vi "MAIN_red.vi"() -> ()   [LabVIEW 2011]
uses:
  <vilib>/event_ctls.llb/eventsource.ctl
  <vilib>/userDefined/High Color/IMAQdx.ctl
  <vilib>/vision/driver/NI_Vision_Acquisition_Software.lvlib
  <vilib>/vision/NI_Vision_Development_Module.lvlib
panel:
  in  "Session In":T1="BW14bits Focused"
  out "X position":dbl
  out "Y position 1":dbl
  out "Y position 2":dbl
  out "X 2":dbl
  out "Source":T2 items=["LabVIEW UI"=0, "ActiveX"=1, "User Event"=25]
  in  "Save":bool
  in  "Color":bool
  out "Image":T3(plugin-control)
  out "Histograph":T4(graph)={"Starting Value"=-32768.0, "Incremental Value"=1.0, "Histogram"=array[65536 elements]}
  out "# Sat. Pixels":sgl(slide) scale=0.0..5000.0
  out "error out 4":errorcluster
  in  "SLM 2":enum32{"Viewer & Positioner", "Hologram Loader"}(tab)
  out "<< CGH_y\n      SLM 2":T3(plugin-control)
  in  "X position 2":dbl(slide)=5.082508250825082 scale=0.0..10.0
  in  "Fine:":dbl(slide)=4.934210526315789 scale=0.0..10.0
  in  "Fine:":dbl(slide)=4.883720930232558 scale=0.0..10.0
  in  "Y position 3":dbl(slide)=4.883720930232558 scale=0.0..10.0
  out "String 2":string
  in  "Xoffset2":dbl=-1325.0
  in  "Yoffset2":dbl=-225.0
  out "String 3":string
  out "SLM 3":T3(plugin-control)
  in  "Radio Buttons":T5(radio)=enum."Radio Selection 2"
  in  "Semi2":bool caption="Boolean"
  in  "Phase correction 2":bool
  in  "M4":bool
  in  "Holo:":dbl=1.0
  out "Ph2 2":dbl
  out "[0 255]":dbl
  out "Ph2":dbl
  in  "Phase:":dbl(slide) scale=0.0..360.0
  out "T2":dbl=100.0
  in  "Trans.:":dbl(slide)=100.0 scale=0.0..100.0
  in  "Active SLM2":bool=TRUE
  in  "SLM 1":enum32{"Viewer & Positioner", "Hologram Loader"}(tab)
  out "CGH_x >>\nSLM 1":T3(plugin-control)
  in  "Y position":dbl(slide)=4.959349593495935 scale=0.0..10.0
  in  "X position 1":dbl(slide)=5.0479233226837055 scale=0.0..10.0
  in  "Fine:":dbl(slide)=5.079872204472843 scale=0.0..10.0
  in  "Fine:":dbl(slide)=5.182186234817814 scale=0.0..10.0
  out "String":string
  in  "Xoffset1":dbl=1300.0
  in  "Yoffset1":dbl=-400.0
  in  "Radio Buttons 2":T5(radio)=enum."Radio Selection 2"
  in  "Semi":bool caption="Boolean"
  in  "Phase correction":bool caption="Amplitude correction"
  in  "M4 2":bool caption="Amplitude correction"
  in  "Holo:":dbl=1.0
  out "Ph1 2":dbl
  out "[0 255]":dbl
  out "Ph1":dbl
  in  "Phase:":dbl(slide) scale=0.0..360.0
  out "T1":dbl=100.0
  in  "Trans.:":dbl(slide)=100.0 scale=0.0..100.0
  out "SLM 2":T3(plugin-control)
  in  "Active SLM1":bool=TRUE
  out "String 4":string
  in  "Parada Total":bool
  out "error out 3":errorcluster
  out "error out 2":errorcluster
  out "error out":errorcluster
  out "path":path
  out "selected path 2":path
  out "selected path":path
  # "BW 14bits"
  # "Y position 2"
  # "Pos. OffSet:"
  # "Y:"
  # "X:"
  # "Arbitrary value settings:"
  # "For gray levels ->"
  # "%"
  # "º"
  # "\\pi rad"
  # "Pos. OffSet:"
  # "X:"
  # "Y:"
  # "Y position 1"
  # "Arbitrary value settings:"
  # "For gray levels ->"
  # "%"
  # "º"
  # "\\pi rad"
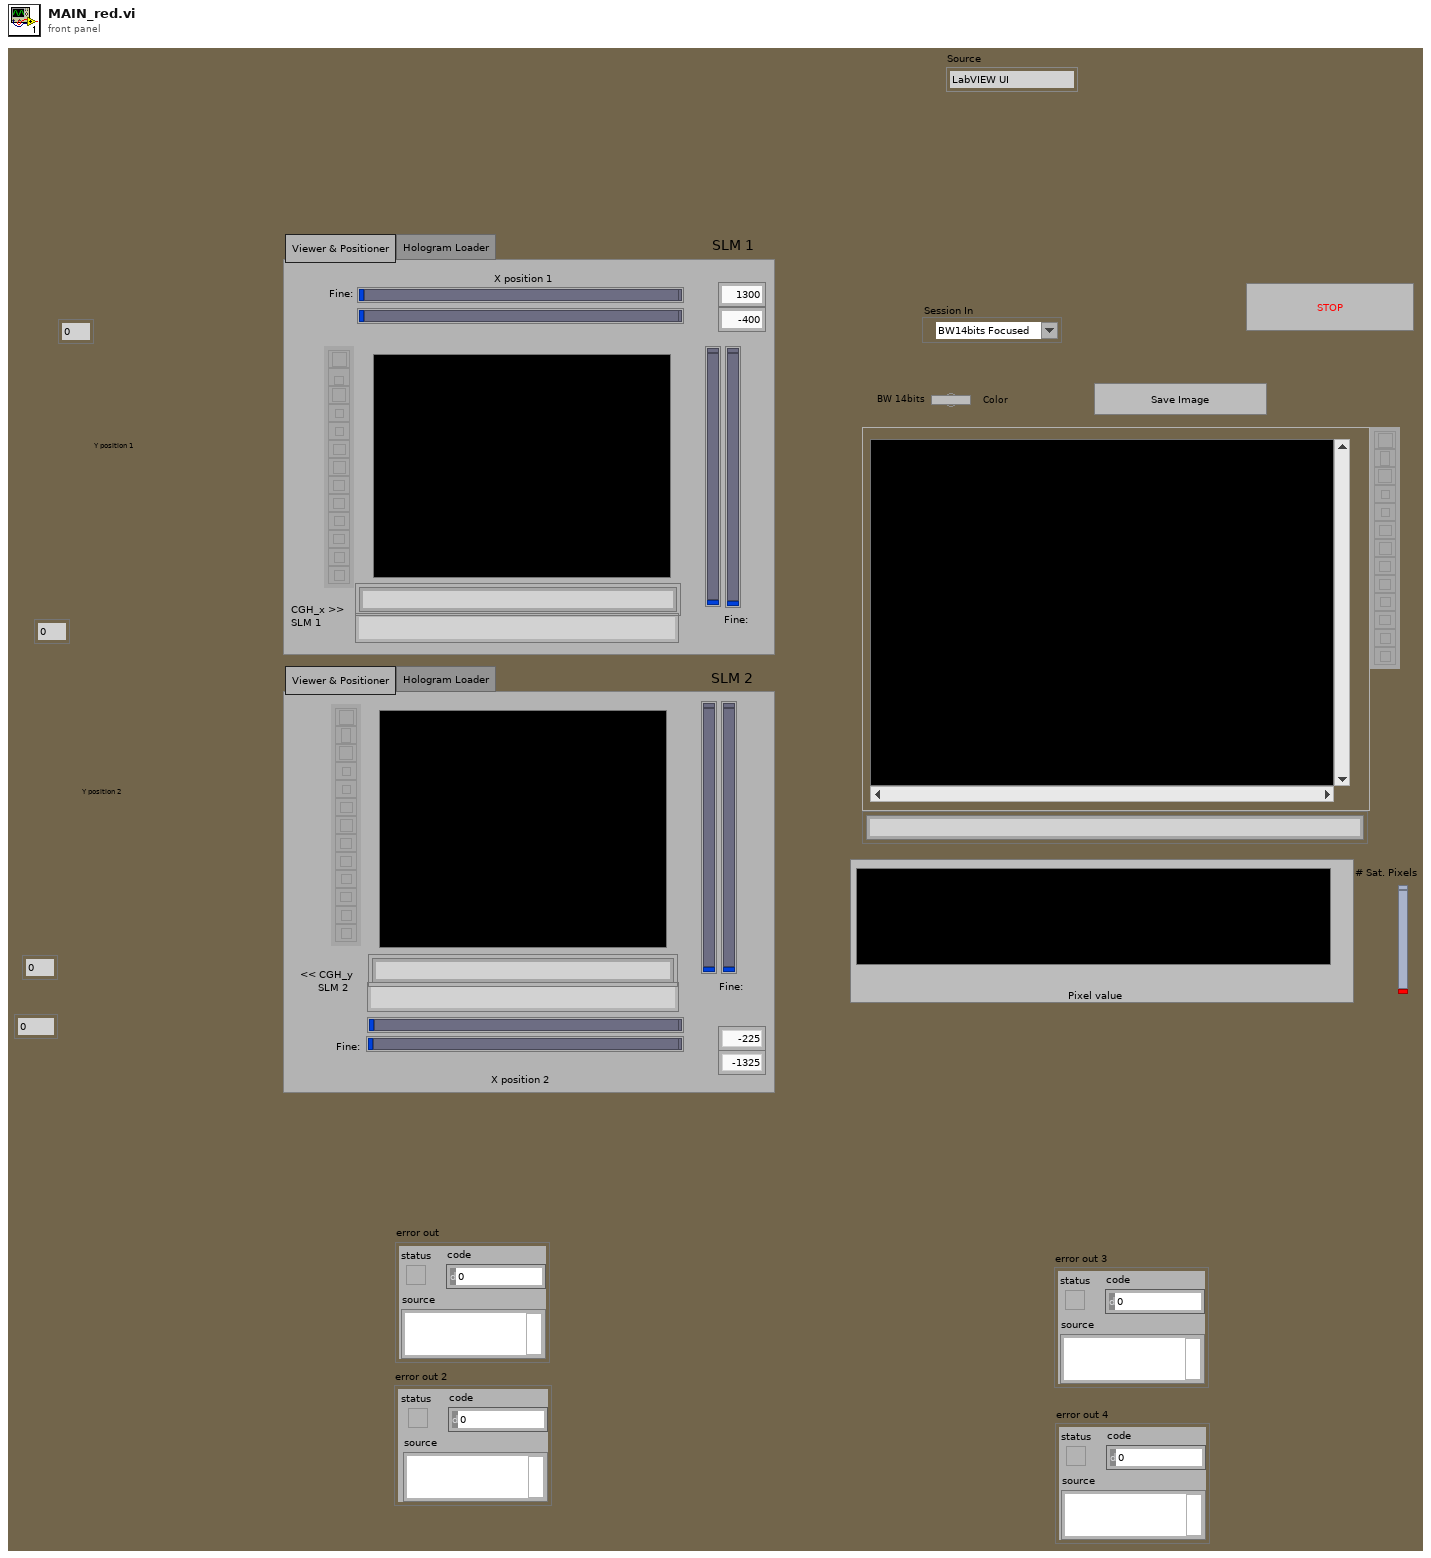
[diagram p1: front panel]
types:
  T1 = typedef "IMAQdx.ctl" = refnum<k21>
  T2 = typedef "eventsource.ctl" = u32
  T3 = typedef "IMAQ Image.ctl" = refnum<image>
  T4 = cluster{"Starting Value":sgl, "Incremental Value":sgl, "Histogram":u32[]}
  T5 = enum32{"Radio Selection 1", "Radio Selection 2", "Radio Selection 3", "Radio Selection 4", "Radio Selection 5", "Radio Selection 6", "Radio Selection 7"}
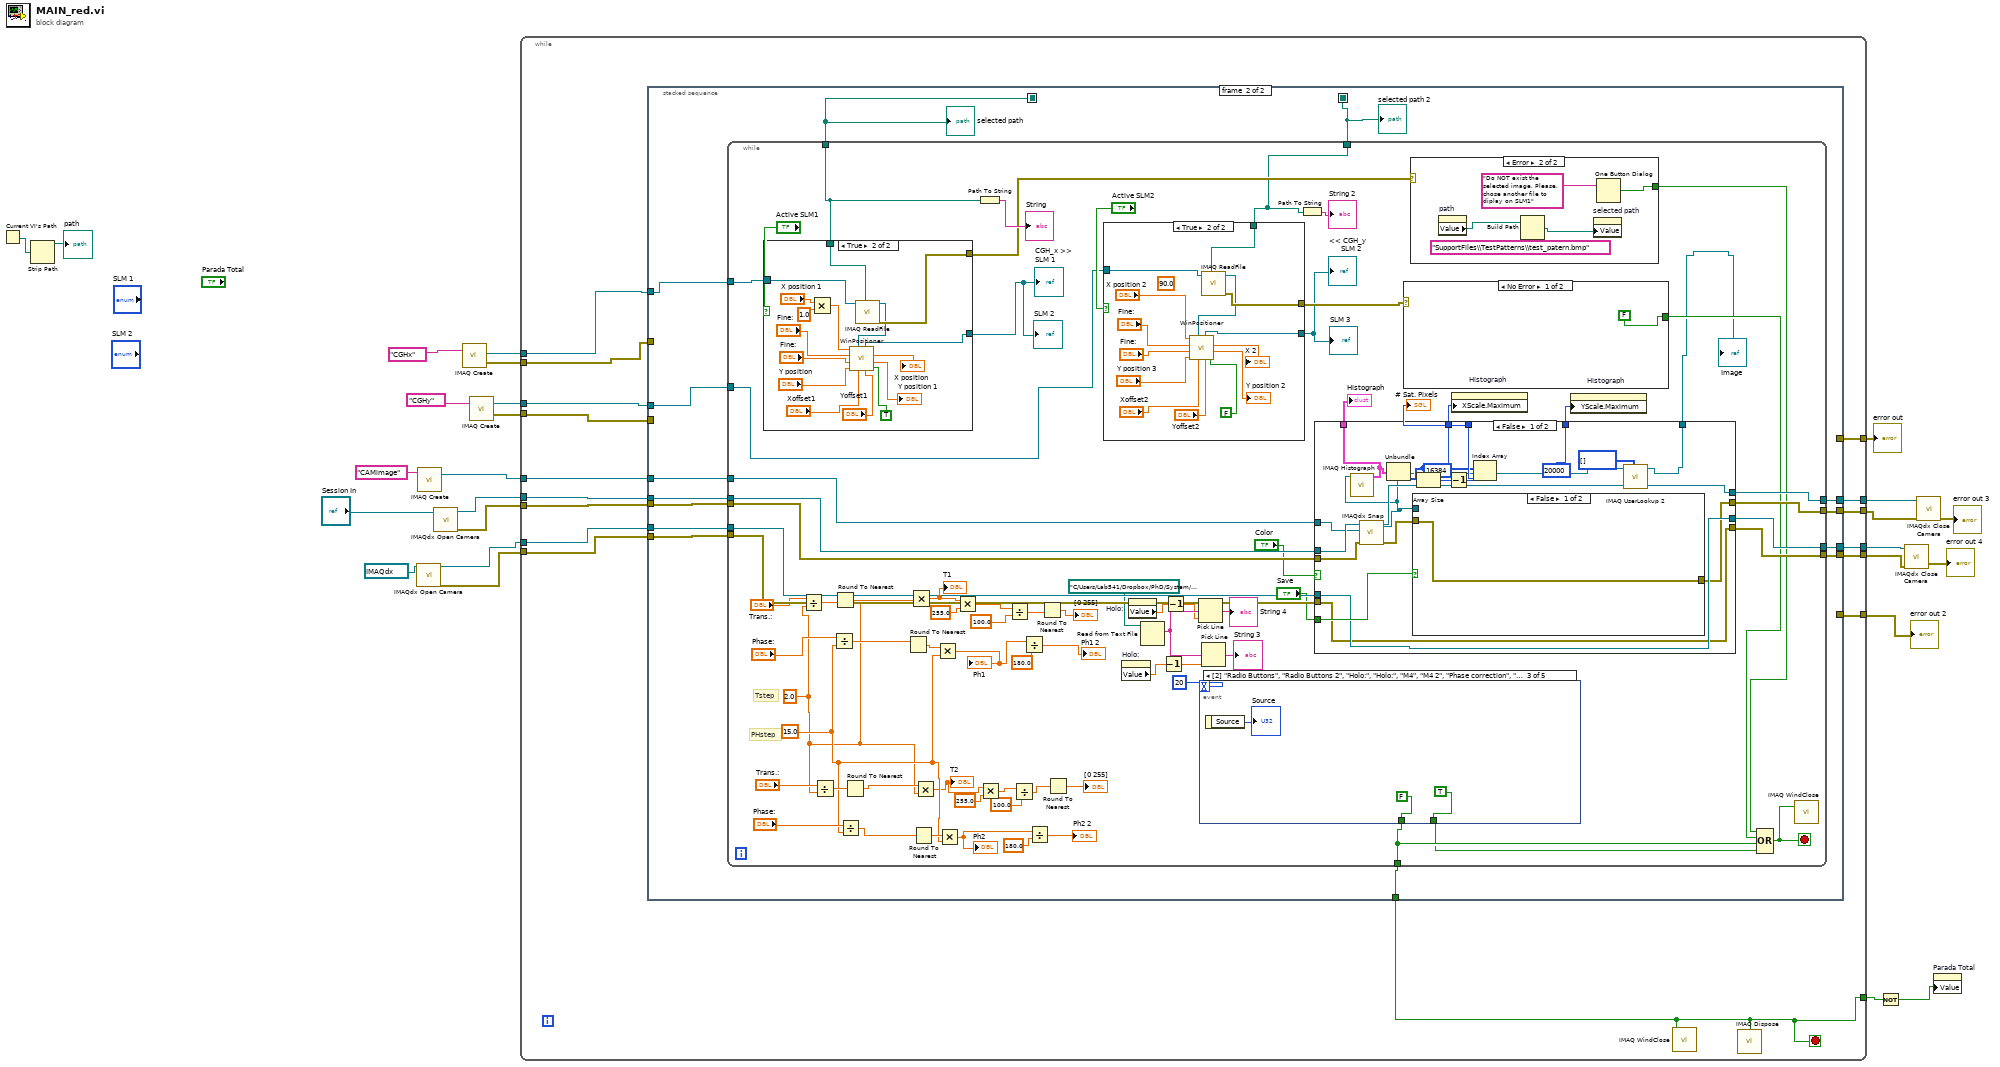
[diagram p0: block diagram]
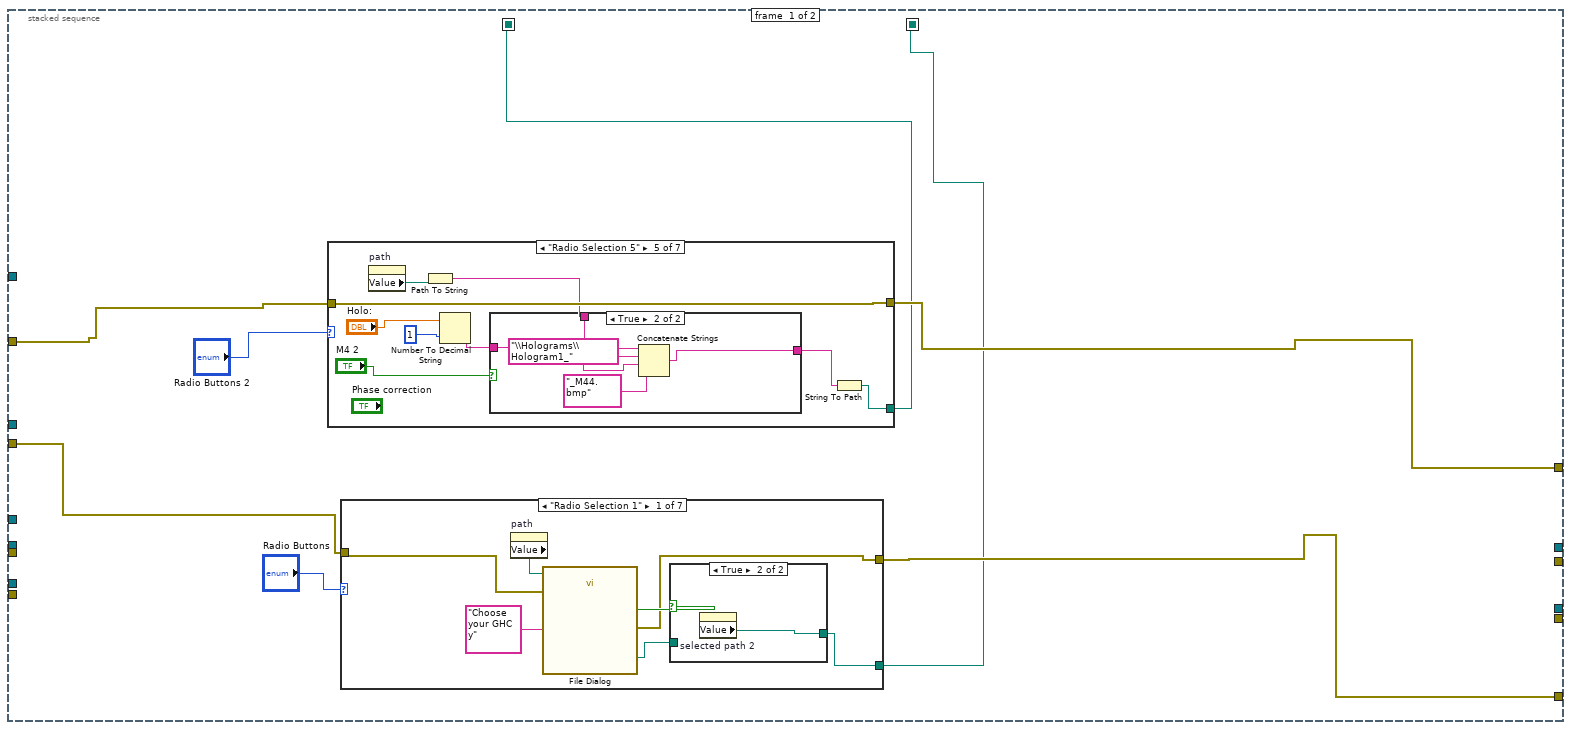
[diagram p2: hidden frame]
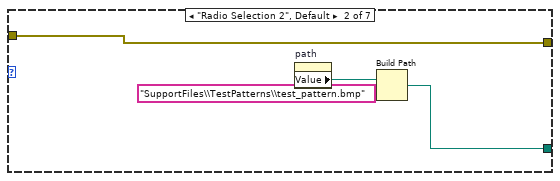
[diagram p4: hidden frame]
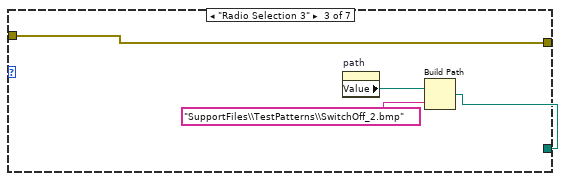
[diagram p5: hidden frame]
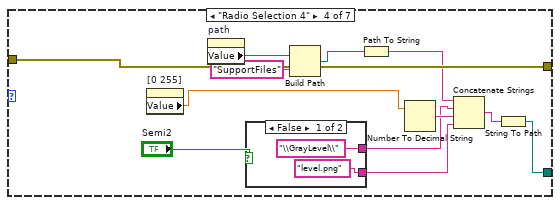
[diagram p6: hidden frame]
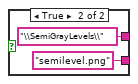
[diagram p7: hidden frame]
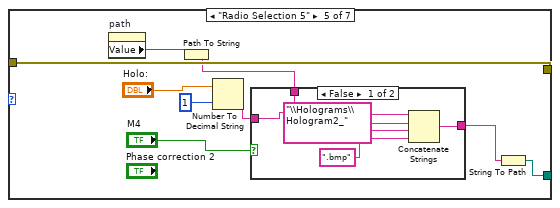
[diagram p8: hidden frame]
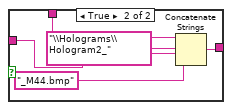
[diagram p9: hidden frame]
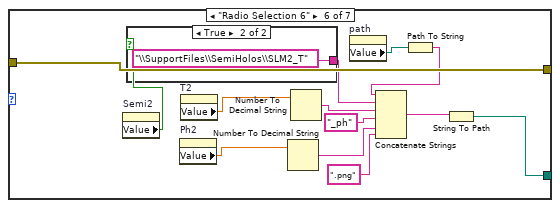
[diagram p10: hidden frame]
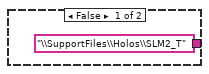
[diagram p11: hidden frame]
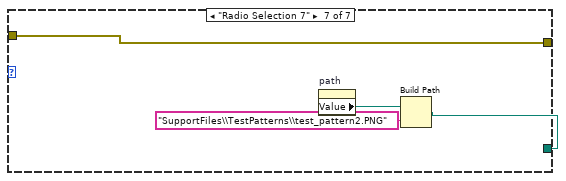
[diagram p12: hidden frame]
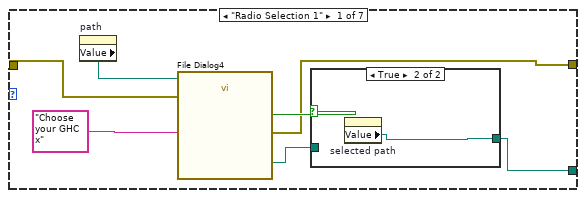
[diagram p13: hidden frame]
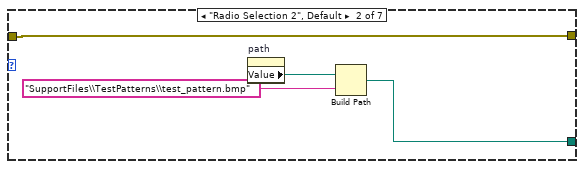
[diagram p15: hidden frame]
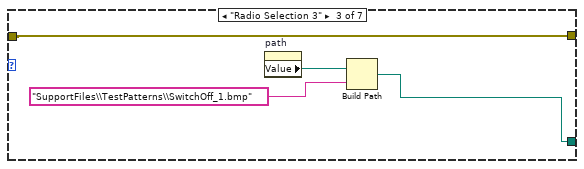
[diagram p16: hidden frame]
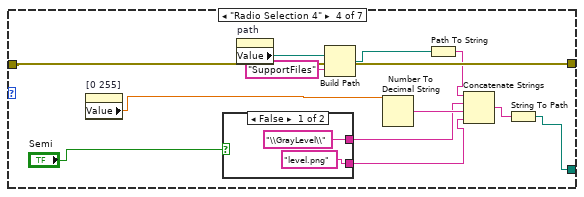
[diagram p17: hidden frame]
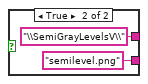
[diagram p18: hidden frame]
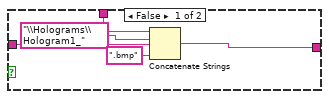
[diagram p19: hidden frame]
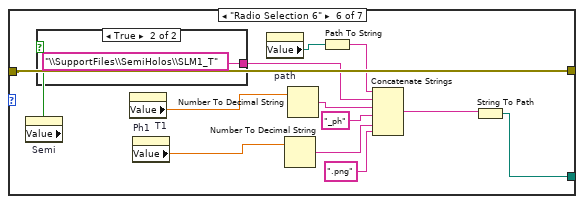
[diagram p20: hidden frame]
diagram:
  n1 = Current VI's Path() -> (path=w20:path)
  n2 = Strip Path(path=w20) -> (stripped path=→"path":path)  [unwired: 1 out]
  n3 = call <vilib>:"IMAQdx Open Camera.vi"("Session In"=T1 "Color") -> ("error out"=w4:errorcluster, "Session Out"=w3:T1)  [unwired: 9 in]
  n4 = call "IMAQ Create"("Image Name"="CAMimage") -> ("New Image"=w16:T3)  [unwired: 4 in, 1 out]
  n5 = call <vilib>:"IMAQdx Open Camera.vi"("Session In"="Session In") -> ("error out"=w2:errorcluster, "Session Out"=w1:T1)  [unwired: 9 in]
  n6 = call "IMAQ Create"("Image Name"="CGHx") -> ("New Image"=w24:T3, "error out"=w21:errorcluster)  [unwired: 4 in]
  n7 = call "IMAQ Create"("Image Name"="CGHy") -> ("New Image"=w23:T3, "error out"=w22:errorcluster)  [unwired: 4 in]
  n8 = while {
    tunnel: w24 -> [w42]
    tunnel: w23 -> [w41]
    tunnel: w22 -> [w40]
    tunnel: [w39] -> w12
    tunnel: w21 -> [w38]
    tunnel: [w37] -> w13
    tunnel: [w27] -> w18
    tunnel: w16 -> [w36]
    tunnel: w1 -> [w35]
    tunnel: w2 -> [w34]
    tunnel: w3 -> [w33]
    tunnel: w4 -> [w32]
    tunnel: [w31] -> w8
    tunnel: [w30] -> w7
    tunnel: [w29] -> w6
    tunnel: [w28] -> w5
    stop <- w27 stop-if-true
    n9 = stacked-sequence {
      seq-local: [w46 _] -> [_ w195]
      seq-local: [w45 _] -> [_ w194]
      tunnel: w42 -> [_ w205]
      tunnel: w41 -> [_ w206]
      tunnel: [_ w193] -> w27
      tunnel: w40 -> [w44 _]
      tunnel: [w50 _] -> w39
      tunnel: w38 -> [w49 _]
      tunnel: [w48 _] -> w37
      tunnel: w36 -> [_ w204]
      tunnel: w35 -> [_ w203]
      tunnel: w34 -> [_ w202]
      tunnel: w33 -> [_ w201]
      tunnel: w32 -> [_ w200]
      tunnel: [_ w199] -> w31
      tunnel: [_ w198] -> w30
      tunnel: [_ w197] -> w29
      tunnel: [_ w196] -> w28
      frame #0 {
        n10 = case shown="\"Radio Selection 5\"" "Radio Buttons 2" {
          tunnel: w49 -> [w124 w134 w138 w150 w163 w186 w192]
          tunnel: [w123 w131 w135 w147 w161 w180 w189] -> w46
          tunnel: [w125 w134 w138 w150 w163 w186 w192] -> w48
          frame "Radio Selection 1" {
            n11 = property on="path" class="Path"() -> ("Value"=w122:path)  [unwired: 2 in, 2 out]
            n12 = call "File Dialog4"("start path"=w122, "prompt"="Choose your GHC x", "error in"=w124) -> ("selected path"=w127:path, "cancelled"=w126:bool, "error out"=w125:errorcluster)  [unwired: 9 in, 1 out]
            n13 = case shown="True" w126 {
              tunnel: [w129 w130] -> w123
              tunnel: w127 -> [w129 _]
              frame False {
              }
              frame True {
                n14 = property on="selected path" class="Path"() -> ("Value"=w130:path)  [unwired: 2 in, 2 out]
              }
            }
          }
          frame "Radio Selection 2", Default {
            n15 = property on="path" class="Path"() -> ("Value"=w133:path)  [unwired: 2 in, 2 out]
            n16 = Build Path(base path=w133, name or relative path="SupportFiles\\TestPatterns\\test_pattern.bmp") -> (appended path=w131:path)
          }
          frame "Radio Selection 3" {
            n17 = property on="path" class="Path"() -> ("Value"=w137:path)  [unwired: 2 in, 2 out]
            n18 = Build Path(base path=w137, name or relative path="SupportFiles\\TestPatterns\\SwitchOff_1.bmp") -> (appended path=w135:path)
          }
          frame "Radio Selection 4" {
            n19 = property on="[0 255]" class="DigNum (strict)"() -> ("Value"=w139:dbl)  [unwired: 2 in, 2 out]
            n20 = case shown="False" "Semi" {
              tunnel: ["\\GrayLevel\\" ("name or relative path") "\\SemiGrayLevelsV\\" ("name or relative path")] -> w141
              tunnel: ["level.png" ("string") "semilevel.png" ("string")] -> w140
              frame False {
              }
              frame True {
              }
            }
            n21 = property on="path" class="Path"() -> ("Value"=w146:path)  [unwired: 2 in, 2 out]
            n22 = Build Path(base path=w146, name or relative path="SupportFiles") -> (appended path=w144:path)
            n23 = Number To Decimal String(number=w139) -> (decimal integer string=w149:string)  [unwired: 1 in]
            n24 = Path To String(path=w144) -> (string=w143:string)
            n25 = Concatenate Strings(w143, w141, w149, w140) -> (w148:string)
            n26 = String To Path(string=w148) -> (path=w147:path)
          }
          frame "Radio Selection 5" {
            n27 = property on="path" class="Path"() -> ("Value"=w157:path)  [unwired: 2 in, 2 out]
            n28 = Path To String(path=w157) -> (string=w156:string)
            n29 = Number To Decimal String(number="Holo:", width (-)=i16 1) -> (decimal integer string=w159:string)
            n30 = case shown="True" "M4 2" {
              tunnel: [w167 w171] -> w162
              tunnel: w159 -> [w166 w170]
              tunnel: w156 -> [w165 w169]
              frame False {
                n31 = Concatenate Strings(w165, "\\Holograms\\Hologram1_" ("string"), w166, ".bmp" ("string")) -> (w167:string)
              }
              frame True {
                n32 = Concatenate Strings(w169, "\\Holograms\\Hologram1_" ("string"), w170, "_M44.bmp" ("string")) -> (w171:string)
              }
            }
            n33 = String To Path(string=w162) -> (path=w161:path)
          }
          frame "Radio Selection 6" {
            n34 = property on="Semi" class="Bool (strict)"() -> ("Value"=w174:bool)  [unwired: 2 in, 2 out]
            n35 = case shown="True" w174 {
              tunnel: ["\\SupportFiles\\Holos\\SLM1_T" ("name or relative path") "\\SupportFiles\\SemiHolos\\SLM1_T" ("name or relative path")] -> w175
              frame False {
              }
              frame True {
              }
            }
            n36 = property on="T1" class="DigNum (strict)"() -> ("Value"=w179:dbl)  [unwired: 2 in, 2 out]
            n37 = property on="Ph1" class="DigNum (strict)"() -> ("Value"=w178:dbl)  [unwired: 2 in, 2 out]
            n38 = property on="path" class="Path"() -> ("Value"=w177:path)  [unwired: 2 in, 2 out]
            n39 = Number To Decimal String(number=w178) -> (decimal integer string=w184:string)  [unwired: 1 in]
            n40 = Number To Decimal String(number=w179) -> (decimal integer string=w185:string)  [unwired: 1 in]
            n41 = Path To String(path=w177) -> (string=w176:string)
            n42 = Concatenate Strings(w176, w175, w185, "_ph" ("Master Thesis (folder)"), w184, ".png" ("Master Thesis (folder)")) -> (w181:string)
            n43 = String To Path(string=w181) -> (path=w180:path)
          }
          frame "Radio Selection 7" {
            n44 = property on="path" class="Path"() -> ("Value"=w191:path)  [unwired: 2 in, 2 out]
            n45 = Build Path(base path=w191, name or relative path="SupportFiles\\TestPatterns\\test_pattern2V.PNG") -> (appended path=w189:path)
          }
        }
        n46 = case shown="\"Radio Selection 1\"" "Radio Buttons" {
          tunnel: w44 -> [w53 w63 w67 w79 w92 w115 w121]
          tunnel: [w52 w60 w64 w76 w90 w109 w118] -> w45
          tunnel: [w54 w63 w67 w79 w92 w115 w121] -> w50
          frame "Radio Selection 1" {
            n47 = property on="path" class="Path"() -> ("Value"=w51:path)  [unwired: 2 in, 2 out]
            n48 = call "File Dialog"("start path"=w51, "prompt"="Choose your GHC y", "error in"=w53) -> ("selected path"=w56:path, "cancelled"=w55:bool, "error out"=w54:errorcluster)  [unwired: 9 in, 1 out]
            n49 = case shown="True" w55 {
              tunnel: [w58 w59] -> w52
              tunnel: w56 -> [w58 _]
              frame False {
              }
              frame True {
                n50 = property on="selected path 2" class="Path"() -> ("Value"=w59:path)  [unwired: 2 in, 2 out]
              }
            }
          }
          frame "Radio Selection 2", Default {
            n51 = property on="path" class="Path"() -> ("Value"=w62:path)  [unwired: 2 in, 2 out]
            n52 = Build Path(base path=w62, name or relative path="SupportFiles\\TestPatterns\\test_pattern.bmp") -> (appended path=w60:path)
          }
          frame "Radio Selection 3" {
            n53 = property on="path" class="Path"() -> ("Value"=w66:path)  [unwired: 2 in, 2 out]
            n54 = Build Path(base path=w66, name or relative path="SupportFiles\\TestPatterns\\SwitchOff_2.bmp") -> (appended path=w64:path)
          }
          frame "Radio Selection 4" {
            n55 = property on="[0 255]" class="DigNum (strict)"() -> ("Value"=w68:dbl)  [unwired: 2 in, 2 out]
            n56 = property on="path" class="Path"() -> ("Value"=w75:path)  [unwired: 2 in, 2 out]
            n57 = case shown="False" "Semi2" {
              tunnel: ["\\GrayLevel\\" ("name or relative path") "\\SemiGrayLevels\\" ("name or relative path")] -> w71
              tunnel: ["level.png" ("string") "semilevel.png" ("string")] -> w70
              frame False {
              }
              frame True {
              }
            }
            n58 = Build Path(base path=w75, name or relative path="SupportFiles") -> (appended path=w73:path)
            n59 = Path To String(path=w73) -> (string=w72:string)
            n60 = Number To Decimal String(number=w68) -> (decimal integer string=w78:string)  [unwired: 1 in]
            n61 = Concatenate Strings(w72, w71, w78, w70) -> (w77:string)
            n62 = String To Path(string=w77) -> (path=w76:path)
          }
          frame "Radio Selection 5" {
            n63 = property on="path" class="Path"() -> ("Value"=w87:path)  [unwired: 2 in, 2 out]
            n64 = Path To String(path=w87) -> (string=w86:string)
            n65 = Number To Decimal String(number="Holo:", width (-)=i16 1) -> (decimal integer string=w85:string)
            n66 = case shown="False" "M4" {
              tunnel: w86 -> [w95 w102]
              tunnel: [w93 w99] -> w91
              tunnel: w85 -> [w96 w100]
              frame False {
                n67 = Concatenate Strings(w95, "\\Holograms\\Hologram2_" ("string"), w96, ".bmp" ("string")) -> (w93:string)
              }
              frame True {
                n68 = Concatenate Strings(w102, "\\Holograms\\Hologram2_" ("string"), w100, "_M44.bmp" ("string")) -> (w99:string)
              }
            }
            n69 = String To Path(string=w91) -> (path=w90:path)
          }
          frame "Radio Selection 6" {
            n70 = property on="Semi2" class="Bool (strict)"() -> ("Value"=w106:bool)  [unwired: 2 in, 2 out]
            n71 = case shown="True" w106 {
              tunnel: ["\\SupportFiles\\Holos\\SLM2_T" ("name or relative path") "\\SupportFiles\\SemiHolos\\SLM2_T" ("name or relative path")] -> w103
              frame False {
              }
              frame True {
              }
            }
            n72 = property on="Ph2" class="DigNum (strict)"() -> ("Value"=w107:dbl)  [unwired: 2 in, 2 out]
            n73 = property on="T2" class="DigNum (strict)"() -> ("Value"=w108:dbl)  [unwired: 2 in, 2 out]
            n74 = Number To Decimal String(number=w107) -> (decimal integer string=w113:string)  [unwired: 1 in]
            n75 = Number To Decimal String(number=w108) -> (decimal integer string=w114:string)  [unwired: 1 in]
            n76 = property on="path" class="Path"() -> ("Value"=w105:path)  [unwired: 2 in, 2 out]
            n77 = Path To String(path=w105) -> (string=w104:string)
            n78 = Concatenate Strings(w104, w103, w114, "_ph" ("Master Thesis (folder)"), w113, ".png" ("Master Thesis (folder)")) -> (w110:string)
            n79 = String To Path(string=w110) -> (path=w109:path)
          }
          frame "Radio Selection 7" {
            n80 = property on="path" class="Path"() -> ("Value"=w120:path)  [unwired: 2 in, 2 out]
            n81 = Build Path(base path=w120, name or relative path="SupportFiles\\TestPatterns\\test_pattern2.PNG") -> (appended path=w118:path)
          }
        }
      }
      frame #1 {
        n82 = while {
          tunnel: [w226] -> w193
          tunnel: w195 -> [w273]
          tunnel: w194 -> [w223]
          tunnel: w206 -> [w227]
          tunnel: w205 -> [w280]
          tunnel: w204 -> [w247]
          tunnel: w203 -> [w246]
          tunnel: w202 -> [w245]
          tunnel: w201 -> [w244]
          tunnel: w200 -> [w243]
          tunnel: [w236] -> w199
          tunnel: [w235] -> w198
          tunnel: [w234] -> w197
          tunnel: [w233] -> w196
          stop <- w248 stop-if-true
          w253 = 15.0 ("x")
          w239 = 2.0 ("x")
          # "PHstep"
          # "Tstep"
          n83 = case shown="True" "Active SLM1" {
            selector: "Active SLM1" -> [w308 _]
            tunnel: w280 -> [w307 w326]
            tunnel: w273 -> [_ w323]
            tunnel: [w306 w311] -> w222
            tunnel: [w309 w322] -> w228
            frame False {
              n84 = property on="path" class="Path"() -> ("Value"=w304:path)  [unwired: 2 in, 2 out]
              n85 = call "IMAQ WindShow"("Hide/Show (Show)"=w308, "Window Number (0...15)"=1) -> ("error out"=w309:errorcluster)  [unwired: 4 in, 2 out]
              n86 = Build Path(base path=w304, name or relative path="SupportFiles\\GrayLevel\\NoImage.png") -> (appended path=w305:path)
              n87 = call "IMAQ ReadFile"("File Path"=w305, "Image"=w307) -> ("Image Out"=w306:T3)  [unwired: 5 in, 4 out]
            }
            frame True {
              n88 = Multiply(x="X position 1", y=1.0 ("x")) -> (x*y=w321:dbl)
              n89 = call "IMAQ ReadFile"("File Path"=w323, "Image"=w326) -> ("error out"=w322:errorcluster, "Image Out"=w312:T3)  [unwired: 5 in, 3 out]
              n90 = call "WinPositioner.vi"("Display?"=TRUE, "Yoffset 2"="Yoffset1", "Xoffset"="Xoffset1", "Image"=w312, "Y position"="Y position", "Fine Y position"="Fine:", "Fine X position"="Fine:", "X position"=w321) -> ("Y position"=→"Y position 1":dbl, "X position"=→"X position":dbl, "CGH_x"=w311:T3)  [unwired: 1 in]
            }
          }
          "CGH_x >>\nSLM 1" <- w222
          "SLM 2" <- w222
          n91 = Divide(x="Trans.:", y=w239) -> (x/y=w272:dbl)
          n92 = Divide(x="Trans.:", y=w239) -> (x/y=w264:dbl)
          n93 = Divide(x="Phase:", y=w253) -> (x/y=w279:dbl)
          n94 = Round To Nearest(number=w272) -> (nearest integer value=w276:dbl)
          n95 = Divide(x="Phase:", y=w253) -> (x/y=w255:dbl)
          n96 = Round To Nearest(number=w264) -> (nearest integer value=w263:dbl)
          n97 = Round To Nearest(number=w279) -> (nearest integer value=w277:dbl)
          n98 = Multiply(x=w276, y=w239) -> (x*y=w271:dbl)
          "T1" <- w271
          n99 = Round To Nearest(number=w255) -> (nearest integer value=w254:dbl)
          n100 = Multiply(x=w263, y=w239) -> (x*y=w252:dbl)
          "T2" <- w252
          n101 = Multiply(x=w277, y=w253) -> (x*y=w265:dbl)
          "Ph1" <- w265
          n102 = Multiply(x=w254, y=w253) -> (x*y=w251:dbl)
          "Ph2" <- w251
          n103 = Multiply(x=w271, y=255.0) -> (x*y=w269:dbl)
          n104 = Path To String(path=w273) -> (string=→"String":string)
          n105 = Multiply(x=w252, y=255.0) -> (x*y=w261:dbl)
          n106 = Divide(x=w269, y=100.0) -> (x/y=w266:dbl)
          n107 = Divide(x=w261, y=100.0) -> (x/y=w259:dbl)
          n108 = Divide(x=w265, y=180.0) -> (x/y=→"Ph1 2":dbl)
          n109 = Divide(x=w251, y=180.0) -> (x/y=→"Ph2 2":dbl)
          n110 = Round To Nearest(number=w266) -> (nearest integer value=→"[0 255]":dbl)
          n111 = Round To Nearest(number=w259) -> (nearest integer value=→"[0 255]":dbl)
          n112 = case shown="True" "Active SLM2" {
            selector: "Active SLM2" -> [w286 _]
            tunnel: w227 -> [w281 w300]
            tunnel: [w282 w290] -> w221
            tunnel: w223 -> [_ w301]
            tunnel: [w288 w302] -> w230
            frame False {
              n113 = property on="path" class="Path"() -> ("Value"=w284:path)  [unwired: 2 in, 2 out]
              n114 = call "IMAQ WindShow"("Hide/Show (Show)"=w286, "Window Number (0...15)"=2) -> ("error out"=w288:errorcluster)  [unwired: 4 in, 2 out]
              n115 = Build Path(base path=w284, name or relative path="SupportFiles\\GrayLevel\\NoImage.png") -> (appended path=w285:path)
              n116 = call "IMAQ ReadFile"("File Path"=w285, "Image"=w281) -> ("Image Out"=w282:T3)  [unwired: 5 in, 4 out]
            }
            frame True {
              (unwired) sgl 90.0 ("Angle (degrees)")
              n117 = call "IMAQ ReadFile"("File Path"=w301, "Image"=w300) -> ("error out"=w302:errorcluster, "Image Out"=w289:T3)  [unwired: 5 in, 3 out]
              n118 = call "WinPositioner.vi"("Display?"=FALSE, "Yoffset 2"="Yoffset2", "Xoffset"="Xoffset2", "Image"=w289, "Y position"="Y position 3", "Fine Y position"="Fine:", "Fine X position"="Fine:", "X position"="X position 2") -> ("Y position"=→"Y position 2":dbl, "X position"=→"X 2":dbl, "CGH_x"=w290:T3)  [unwired: 1 in]
            }
          }
          "<< CGH_y\n      SLM 2" <- w221
          "SLM 3" <- w221
          n119 = property on="Holo:" class="DigNum (strict)"() -> ("Value"=w212:dbl)  [unwired: 2 in, 2 out]
          n120 = property on="Holo:" class="DigNum (strict)"() -> ("Value"=w214:dbl)  [unwired: 2 in, 2 out]
          n121 = Read from Text File(file (use dialog)=path "C:/Users/Lab541/Dropbox/PhD/System/+scripts/design_kinds.txt") -> (text=w215:string)  [unwired: 3 in, 3 out]
          n122 = Decrement(x=w212) -> (x-1=w211:dbl)
          n123 = Decrement(x=w214) -> (x-1=w213:dbl)
          n124 = Pick Line(multi-line string=w215, line index=w213) -> (output string=→"String 4":string)  [unwired: 1 in]
          n125 = event shown="[2] \"Radio Buttons\", \"Radio Buttons 2\", \"Holo:\", \"Holo:\", \"M4\", \"M4 2\", \"Phase correction\", \"Phase correction 2\", \"Semi\", \"Semi2\": Value Change;  \"Trans.:\", \"Phase:\", \"Trans.:\", \"Phase:\": Mouse Up" {
            selector: _ -> [_ _ _ _ _]
            dyn-events: _ -> [_ _ _ _ _]
            timeout: 20 -> [_ _ _ _ _]
            tunnel: [w327 TRUE ("value") TRUE ("value") w333 w336] -> w225
            tunnel: [w327 w328 FALSE ("NewVal") w333 w336] -> w226
            event Timeout {
              w327 = FALSE ("NewVal")
              n126 = event-data() -> ()  [unwired: 1 in, 2 out]
            }
            event "Parada Total": Value Change {
              n127 = event-data() -> ("NewVal"=w328:bool)  [unwired: 1 in]
            }
            event "Radio Buttons", "Radio Buttons 2", "Holo:", "Holo:", "M4", "M4 2", "Phase correction", "Phase correction 2", "Semi", "Semi2": Value Change; "Trans.:", "Phase:", "Trans.:", "Phase:": Mouse Up {
              n128 = event-data() -> ("Source"=→"Source":T2)  [unwired: 1 in]
            }
            event "Active SLM1": Value Change {
              w333 = FALSE ("NewVal")
              n129 = event-data() -> ("NewVal"=w335:bool)  [unwired: 1 in]
              n130 = call "IMAQ WindShow"("Hide/Show (Show)"=w335, "Window Number (0...15)"=1) -> ()  [unwired: 4 in, 3 out]
            }
            event "Active SLM2": Value Change {
              w336 = FALSE ("NewVal")
              n131 = event-data() -> ("NewVal"=w337:bool)  [unwired: 1 in]
              n132 = call "IMAQ WindShow"("Hide/Show (Show)"=w337, "Window Number (0...15)"=2) -> ()  [unwired: 4 in, 3 out]
            }
          }
          n133 = Pick Line(multi-line string=w215, line index=w211) -> (output string=→"String 3":string)  [unwired: 1 in]
          n134 = Path To String(path=w223) -> (string=→"String 2":string)
          n135 = case shown="False" "Color" {
            tunnel: "Save" -> [w355 w385]
            tunnel: [w353 w388] -> w233
            tunnel: [w340 w379] -> w207
            tunnel: w247 -> [w349 w383]
            tunnel: w246 -> [w351 w381]
            tunnel: w245 -> [w350 w380]
            tunnel: w244 -> [w354 w382]
            tunnel: w243 -> [w353 w384]
            tunnel: [w354 w386] -> w234
            tunnel: [w356 w381] -> w236
            tunnel: [w352 w380] -> w235
            tunnel: [w348 w371] -> w220
            tunnel: [w347 w378] -> w219
            tunnel: [16384 768] -> w218
            tunnel: [20000 200000] -> w217
            frame False {
              n136 = call <vilib>:"IMAQdx Snap.vi"("error in"=w350, "Image In"=w349, "Session In"=w351) -> ("error out"=w357:errorcluster, "Image Out"=w341:T3, "Session Out"=w356:T1)  [unwired: 6 in]
              n137 = call "IMAQ Histograph"("Image"=w341) -> ("Histogram Graph"=w348:T4)  [unwired: 7 in, 3 out]
              n138 = Unbundle(w348) -> ("Histogram"=w346:u32[])  [unwired: 2 out]
              n139 = case shown="False" w355 {
                tunnel: [w358 w361] -> w352
                tunnel: w341 -> [_ w359]
                tunnel: w357 -> [w358 w360]
                frame False {
                }
                frame True {
                  n140 = property on="path" class="Path"() -> ("Value"=w369:path)  [unwired: 2 in, 2 out]
                  n141 = Build Path(base path=w369, name or relative path="Images") -> (appended path=w368:path)
                  n142 = call "File Dialog3"("start path"=w368, "prompt"="Save image", "button label"="Save", "error in"=w360, "pattern (all files)"=".png", "pattern label"="PNG") -> ("selected path"=w370:path, "error out"=w362:errorcluster)  [unwired: 6 in, 2 out]
                  n143 = call-poly "IMAQ Write File 2"("error in (no error)"=w362, "File Path"=w370, "Image"=w359) -> ("error out"=w361:errorcluster)  [unwired: 7 in, 1 out]
                }
              }
              n144 = Array Size(array=w346) -> (size(s)=w345:i32)
              n145 = Decrement(x=w345) -> (x-1=w344:i32)
              n146 = Index Array(array=w346, index=w344) -> (element=w347:u32)
              n147 = call "IMAQ UserLookup 2"("Image Src"=w341, "Lookup Table"=i32[] []) -> ("Image Dst Out"=w340:T3)  [unwired: 5 in, 1 out]
            }
            frame True {
              n148 = call <vilib>:"IMAQdx Snap.vi"("error in"=w384, "Image In"=w383, "Session In"=w382) -> ("error out"=w387:errorcluster, "Image Out"=w379:T3, "Session Out"=w386:T1)  [unwired: 6 in]
              n149 = case shown="True" TRUE {
                tunnel: w379 -> [w390 w395]
                tunnel: [w389 w391] -> w371
                frame False {
                  n150 = call "IMAQ Histograph"("Image"=w390) -> ("Histogram Graph"=w389:T4)  [unwired: 7 in, 3 out]
                }
                frame True {
                  n151 = call "IMAQ ColorHistograph"("Image Src"=w395) -> ("Red or Hue Histogram Graph"=w394:T4, "Green or Sat Histogram Graph"=w393:T4, "Blue or Luma or Val or Inten Histogram Graph"=w392:T4)  [unwired: 5 in, 1 out]
                  n152 = Compound Arithmetic op=ADD(w394, w393, w392) -> (w391:T4)
                }
              }
              n153 = Unbundle(w371) -> ("Histogram"=w377:u32[])  [unwired: 2 out]
              n154 = case shown="True" w385 {
                tunnel: [w396 w406] -> w388
                tunnel: w379 -> [_ w397]
                tunnel: w387 -> [w396 w398]
                frame False {
                }
                frame True {
                  n155 = property on="path" class="Path"() -> ("Value"=w405:path)  [unwired: 2 in, 2 out]
                  n156 = Build Path(base path=w405, name or relative path="Images") -> (appended path=w404:path)
                  n157 = call "File Dialog2"("start path"=w404, "prompt"="Save image", "button label"="Save", "error in"=w398, "pattern (all files)"=".png", "pattern label"="PNG") -> ("selected path"=w408:path, "error out"=w407:errorcluster)  [unwired: 6 in, 2 out]
                  n158 = call-poly "IMAQ Write File 2"("error in (no error)"=w407, "File Path"=w408, "Image"=w397) -> ("error out"=w406:errorcluster)  [unwired: 7 in, 1 out]
                }
              }
              n159 = Array Size(array=w377) -> (size(s)=w376:i32)
              n160 = Decrement(x=w376) -> (x-1=w375:i32)
              n161 = Index Array(array=w377, index=w375) -> (element=w378:u32)
            }
          }
          "Image" <- w207
          "Histograph" <- w220
          "# Sat. Pixels" <- w219
          n162 = case shown="No Error" w230 {
            tunnel: [FALSE ("true") w410] -> w231
            frame No Error {
            }
            frame Error {
              n163 = property on="path" class="Path"() -> ("Value"=w414:path)  [unwired: 2 in, 2 out]
              n164 = Build Path(base path=w414, name or relative path="SupportFiles\\TestPatterns\\test_patern.bmp") -> (appended path=w413:path)
              n165 = property on="selected path 2" class="Path"("Value"=w413) -> ()  [unwired: 2 in, 2 out]
              n166 = One Button Dialog(message="Do NOT exist the selected image. Please, chose another file to diplay on SLM2") -> (true=w410:bool)  [unwired: 1 in]
            }
          }
          n167 = case shown="Error" w228 {
            tunnel: [FALSE ("true") w418] -> w232
            frame No Error {
            }
            frame Error {
              n168 = property on="path" class="Path"() -> ("Value"=w416:path)  [unwired: 2 in, 2 out]
              n169 = Build Path(base path=w416, name or relative path="SupportFiles\\TestPatterns\\test_patern.bmp") -> (appended path=w419:path)
              n170 = property on="selected path" class="Path"("Value"=w419) -> ()  [unwired: 2 in, 2 out]
              n171 = One Button Dialog(message="Do NOT exist the selected image. Please, chose another file to diplay on SLM1") -> (true=w418:bool)  [unwired: 1 in]
            }
          }
          n172 = property on="Histograph" class="WFGraph (strict)"("XScale.Maximum"=w218) -> ()  [unwired: 2 in, 2 out]
          n173 = property on="Histograph" class="WFGraph (strict)"("YScale.Maximum"=w217) -> ()  [unwired: 2 in, 2 out]
          n174 = Compound Arithmetic op=OR(w232, w231, w226, w225) -> (w248:bool)
          n175 = call "IMAQ WindClose"("Close All Windows (False)"=w248) -> ()  [unwired: 5 in, 1 out]
        }
        "selected path" <- w195
        "selected path 2" <- w194
      }
    }
    n176 = call "IMAQ WindClose"("Close All Windows (False)"=w27) -> ()  [unwired: 5 in, 1 out]
    n177 = call "IMAQ Dispose"("All Images? (No)"=w27) -> ()  [unwired: 5 in, 1 out]
  }
  "error out" <- w13
  "error out 2" <- w12
  n178 = Not(x=w18) -> (.not. x?=w11:bool)
  n179 = call <vilib>:"IMAQdx Close Camera.vi"("error in"=w5, "Session In"=w6) -> ("error out"=→"error out 4":errorcluster)  [unwired: 9 in]
  n180 = call <vilib>:"IMAQdx Close Camera.vi"("error in"=w7, "Session In"=w8) -> ("error out"=→"error out 3":errorcluster)  [unwired: 9 in]
  n181 = property on="Parada Total" class="Bool (strict)"("Value"=w11) -> ()  [unwired: 2 in, 2 out]
